vi "2016 Shooter Controller.vi"(8 "error in":errorcluster) -> ()   [LabVIEW 2016]
doc: "This VI executes continuously carrying out the current operation and responding to updates or new operations. It will often contain the timing or control code that is difficult to place directly in TeleOp. This VI generally opens all sensors and motors and isolates the rest of the robot code from knowing how the operations are carried out."
uses:
  2016 Shooter Setpoints.ctl
  2016 Shooter Operations.ctl
  <vilib>/Rock Robotics/WPI/ThirdParty/CanMotor/TalonSRX/WPI_CANTalonSRX_APIControlMode.ctl
  <vilib>/Rock Robotics/WPI/Solenoid/WPI_SolenoidChannel.ctl
  <vilib>/Rock Robotics/WPI/Solenoid/WPI_SolenoidOpenSingle.vi
panel:
  out "Current\nCmd":string
  # "Tip: It may be helpful to observe inputs and sensor values.\nYou may also want to display tuning or debugging controls."
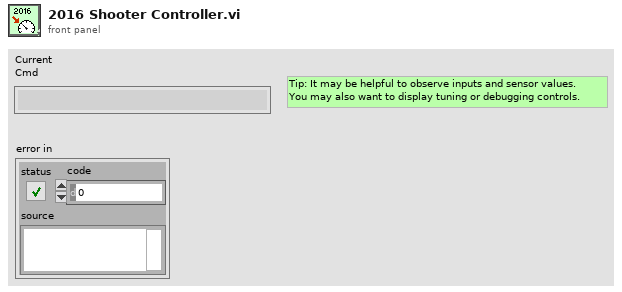
[diagram p1: front panel]
types:
  T1 = typedef "WPI_SolenoidChannel.ctl" = enum8{"Solenoid 0", "Solenoid 1", "Solenoid 2", "Solenoid 3", "Solenoid 4", "Solenoid 5", "Solenoid 6", "Solenoid 7", "Invalid"}
  T2 = typedef "WPI_CANTalonSRX_APIControlMode.ctl" = enum8{"Percent VBus", "Speed", "Position", "Slave", "Unchanged / Invalid", "Voltage Compensation", "Current", "Motion Profile", "Motion Magic"}
  T3 = typedef "2016 Shooter Setpoints.ctl" = cluster{"Operation":T4, "Setpoint":dbl, "Duration":dbl}
  T4 = typedef "2016 Shooter Operations.ctl" = enum16{"Reserve", "Read Current", "Immediate", "Shoot", "Retrieve"}
  T5 = typedef "WPI_MotorControlDeviceRef.ctl" = cluster{"DeviceStatus":errorcluster, "Type":T6, "PWM":cluster{"PWM Channel":T7, "DeadBand":T8}, "CAN":cluster{"Device Number":u8, "SetOutput VI Ref":variant, "GetOutput VI Ref":variant, "Enable VI Ref":variant, "Disable VI Ref":variant, "Data":variant}, "Invert":bool}
  T6 = typedef "WPI_MotorControlType.ctl" = enum16{"PWM", "CAN"}
  T7 = typedef "FPGA_DIOPWMChannel.ctl" = enum8{"PWM 0", "PWM 1", "PWM 2", "PWM 3", "PWM 4", "PWM 5", "PWM 6", "PWM 7", "PWM 8", "PWM 9", "PWM MXP 0", "PWM MXP 1", "PWM MXP 2", "PWM MXP 3", "PWM MXP 4", "PWM MXP 5", "PWM MXP 6", "PWM MXP 7", "PWM MXP 8", "PWM MXP 9", "Invalid"}
  T8 = typedef "WPI_PWMDeadband.ctl" = cluster{"Name":string, "maxPositivePwm":i32, "minPositivePwm":i32, "centerPwm":i32, "maxNegativePwm":i32, "minNegativePwm":i32, "angularRange":u16}
  T9 = typedef "WPI_SolenoidDevRef.ctl" = cluster{"DevStatus":errorcluster, "Pneumatics Control Module":u8, "Forward Solenoid Channel":T1, "Reverse Solenoid Channel":T1}
  T10 = typedef "Command Status Info.ctl" = cluster{"Name":string, "Status":T11, "notifier out":T12}
  T11 = typedef "Completion Status.ctl" = enum16{"Successful", "Aborted", "Incomplete"}
  T12 = typedef "Completion Notifier.ctl" = refnum<notifier>
  T13 = cluster{"Default Command":T3, "Command Timing":cluster{"Start Time (ms)":u32, "Iterations":i32}, "Command Arguments":cluster{"Command Info":T10, "Description":string, "Default Command":T3, "notifier out":refnum<notifier>, "Subsystem Name":string}}
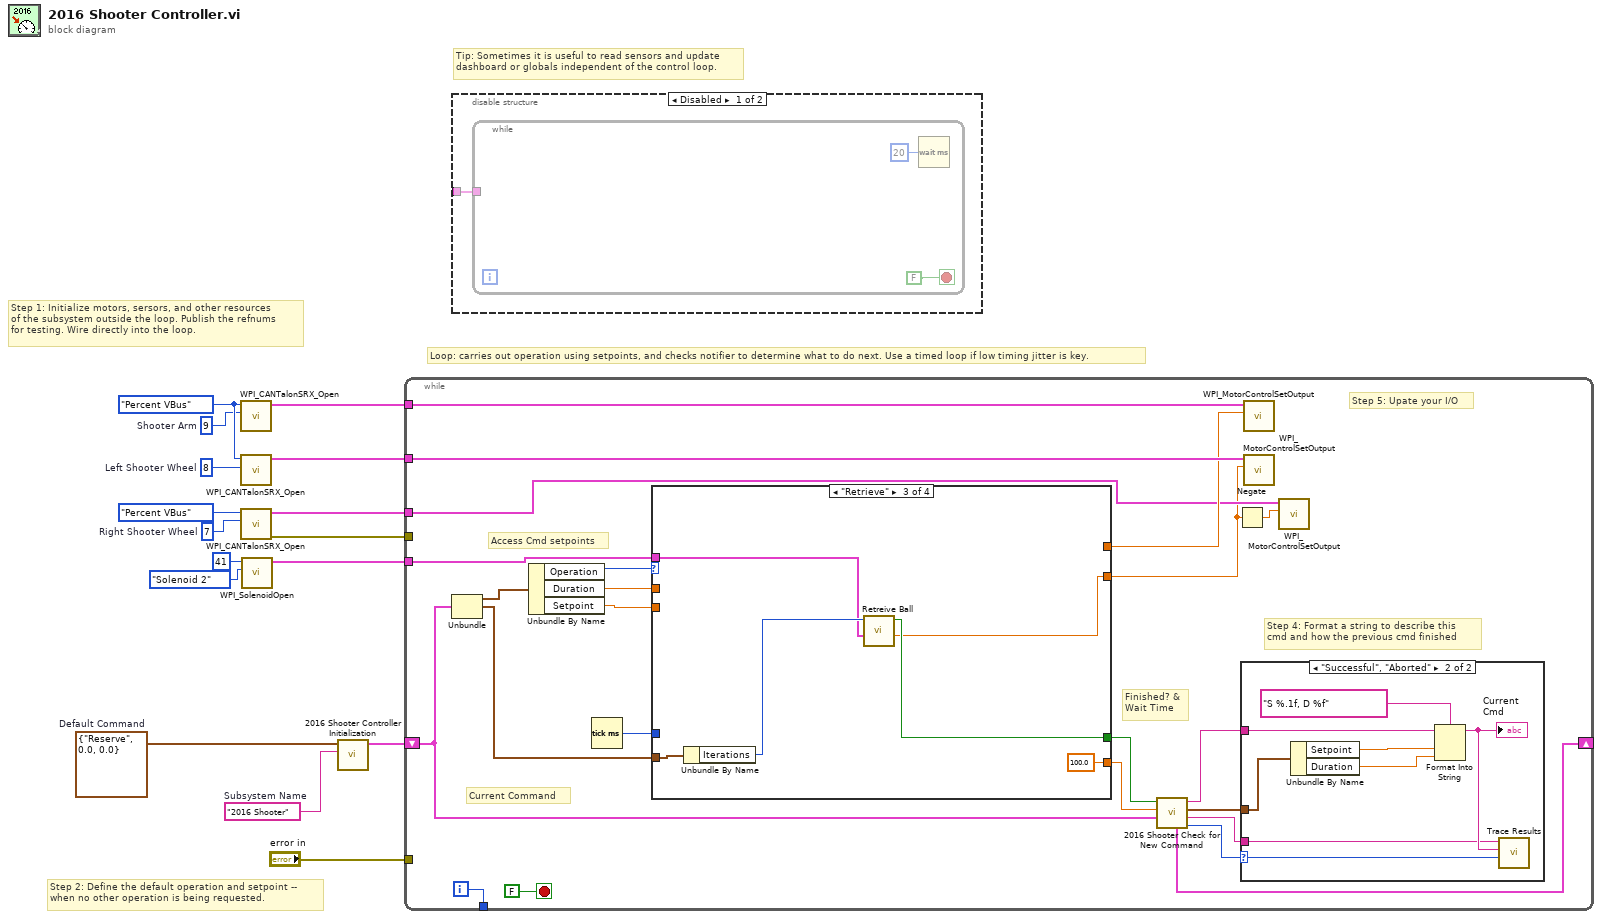
[diagram p0: block diagram]
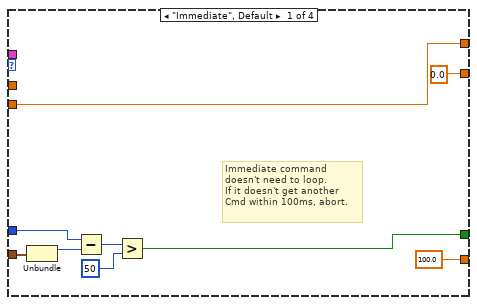
[diagram p4: hidden frame]
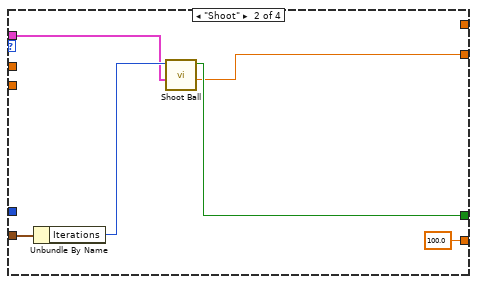
[diagram p5: hidden frame]
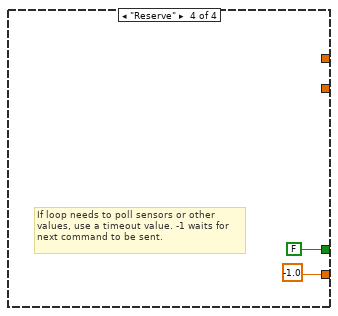
[diagram p6: hidden frame]
diagram:
  w6 = u8 7  # Right Shooter Wheel
  w7 = u8 8  # Left Shooter Wheel
  w8 = u8 9  # Shooter Arm
  w10 = WPI_CANTalonSRX_APIControlMode."Percent VBus" ("Control Mode")
  w13 = T3 {"Operation"=enum."Reserve", "Setpoint"=0.0, "Duration"=0.0}  # Default Command
  w14 = "2016 Shooter"  # Subsystem Name
  # "Tip: Sometimes it is useful to read sensors and update\ndashboard or globals independent of the control loop."
  # "Step 2: Define the default operation and setpoint --\nwhen no other operation is being requested."
  # "Step 1: Initialize motors, sersors, and other resources\nof the subsystem outside the loop. Publish the refnums\nfor testing. Wire directly into the loop."
  # "Loop: carries out operation using setpoints, and checks notifier to determine what to do next. Use a timed loop if low timing jitter is key."
  n1 = call <vilib>:"WPI_CANTalonSRX_Open.vi"("Device Number"=w8, "Control Mode"=w10) -> ("CAN Talon SRX Ref"=w12:T5)  [unwired: 8 in, 1 out]
  n2 = call <vilib>:"WPI_CANTalonSRX_Open.vi"("Device Number"=w7, "Control Mode"=w10) -> ("CAN Talon SRX Ref"=w11:T5)  [unwired: 8 in, 1 out]
  n3 = call <vilib>:"WPI_CANTalonSRX_Open.vi"("Device Number"=w6, "Control Mode"=WPI_CANTalonSRX_APIControlMode."Percent VBus") -> ("error out"=w5:errorcluster, "CAN Talon SRX Ref"=w1:T5)  [unwired: 8 in]
  n4 = call-poly <vilib>:"WPI_SolenoidOpen.vi"("Solenoid Channel"=WPI_SolenoidChannel."Solenoid 2", "Pneumatics Control Module (0)"=u8 41) -> ("SolenoidDevRef"=w2:T9)  [unwired: 8 in, 1 out]
  n5 = call "2016 Shooter Controller Initialization.vi"("Subsystem Name"=w14, "Default Command"=w13) -> ("Command Info"=w15:T13)  [unwired: 9 in]
  n6 = while {
    shift-right: [w30] -> _
    shift-left: w15 -> [w31]
    tunnel: [w38] -> _
    tunnel: "error in" -> [_]
    tunnel: w12 -> [w23]
    tunnel: w11 -> [w22]
    tunnel: w5 -> [_]
    tunnel: w2 -> [w20]
    tunnel: w1 -> [w19]
    i -> [w38]
    stop <- FALSE stop-if-true
    # "Step 5: Upate your I/O"
    # "Step 4: Format a string to describe this\ncmd and how the previous cmd finished"
    # "Current Command"
    # "Access Cmd setpoints"
    # "Finished? &\nWait Time"
    n7 = Unbundle(w31) -> ("Default Command"=w37:T3, "Command Timing"=w33:cluster{"Start Time (ms)":u32, "Iterations":i32})  [unwired: 1 out]
    n8 = Unbundle By Name(w37) -> ("Operation"=w36:T4, "Duration"=w35:dbl, "Setpoint"=w32:dbl)
    n9 = Tick Count (ms)() -> (millisecond timer value=w34:u32)
    n10 = case shown="\"Retrieve\"" w36 {
      tunnel: [100.0 100.0 100.0 -1.0] -> w28
      tunnel: [w50 w59 w65 FALSE ("ignore previous (F)")] -> w29
      tunnel: w33 -> [w52 w62 w68 _]
      tunnel: w35 -> [_ _ _ _]
      tunnel: w34 -> [w51 _ _ _]
      tunnel: w32 -> [w49 _ _ _]
      tunnel: [0.0 w57 w64 _] -> w18
      tunnel: [w49 _ _ _] -> w21
      tunnel: w20 -> [_ w60 w66 _]
      frame "Immediate", Default {
        # "Immediate command\ndoesn't need to loop.\nIf it doesn't get another\nCmd within 100ms, abort."
        n11 = Unbundle(w52) -> ("Start Time (ms)"=w55:u32)  [unwired: 1 out]
        n12 = Subtract(x=w51, y=w55) -> (x-y=w54:u32)
        n13 = Greater?(x=w54, y=u8 50 ("Left Motor")) -> (0:w50:bool)
      }
      frame "Shoot" {
        n14 = Unbundle By Name(w62) -> ("Iterations"=w61:i32)
        n15 = call "Shoot Ball.vi"("SolenoidDevRef"=w60, "Iteration"=w61) -> ("Speed"=w57:dbl, "Finished"=w59:bool)  [unwired: 8 in]
      }
      frame "Retrieve" {
        n16 = Unbundle By Name(w68) -> ("Iterations"=w67:i32)
        n17 = call "Retreive Ball.vi"("SolenoidDevRef"=w66, "Iteration"=w67) -> ("Speed"=w64:dbl, "Finished"=w65:bool)  [unwired: 8 in]
      }
      frame "Reserve" {
        # "If loop needs to poll sensors or other\nvalues, use a timeout value. -1 waits for\nnext command to be sent."
      }
    }
    n18 = call "2016 Shooter Check for New Command.vi"("Current Command"=w31, "Wait time (ms)"=w28, "Finished?"=w29) -> ("Completion"=w24:T11, "Subsystem Name"=w25:string, "Current Command"=w26:T3, "Initial Trace String"=w27:string, "NextCommand"=w30:T13)  [unwired: 4 in]
    n19 = Negate(x=w18) -> (-x=w17:dbl)
    n20 = case shown="\"Successful\", \"Aborted\"" w24 {
      selector: w24 -> [_ w47]
      tunnel: w27 -> [_ w43]
      tunnel: w26 -> [_ w44]
      tunnel: w25 -> [_ w40]
      frame "Incomplete", Default {
        # "Continuing current command"
      }
      frame "Successful", "Aborted" {
        # "Report and setup for next command"
        n21 = Unbundle By Name(w44) -> ("Setpoint"=w46:dbl, "Duration"=w41:dbl)
        n22 = Format Into String(format string="S %.1f, D %f", initial string=w43, w46, w41) -> (resulting string=w42:string)  [unwired: 1 in, 1 out]
        "Current\nCmd" <- w42
        n23 = call <vilib>:"Trace Results.vi"("Status of previous command"=w47, "Description"=w42, "Subsystem"=w40) -> ()  [unwired: 9 in]
      }
    }
    n24 = call <vilib>:"WPI_MotorControlSetOutput.vi"("Output"=w21, "MotorControlDevRef"=w23) -> ()  [unwired: 7 in, 3 out]
    n25 = call <vilib>:"WPI_MotorControlSetOutput.vi"("Output"=w18, "MotorControlDevRef"=w22) -> ()  [unwired: 7 in, 3 out]
    n26 = call <vilib>:"WPI_MotorControlSetOutput.vi"("Output"=w17, "MotorControlDevRef"=w19) -> ()  [unwired: 7 in, 3 out]
  }
  n27 = disable-structure shown="Disabled" {
    disable-tunnel: _ -> [w71 _]
    frame Disabled {
      n28 = while {
        tunnel: w71 -> [_]
        stop <- FALSE stop-if-true
        n29 = Wait (ms)(milliseconds to wait=u32 20) -> ()  [unwired: 1 out]
      }
    }
    frame Enabled {
    }
  }
